vi "Open Running VI MHLC.vi"(8 "error in (no error)":errorcluster, 10 "Data in":variant, 11 "AppMgr in":refnum<class "Application Manager.lvclass">) -> (0 "error out":errorcluster, 3 "AppMgr out":refnum<class "Application Manager.lvclass">)   [LabVIEW 2017, in "Application Manager.lvclass"]
doc: "Open the Front Panel of the Main VI of the selected Worker's running clone"
uses:
  Application Manager.lvclass
  rqp_Open Running VI.ctl
  Common VIs/DC_UID.ctl
  Application Manager.lvclass/Application Manager.ctl
  rsp_Show Worker Block Diagram.ctl
  <vilib>/Utility/error.llb/Error Cluster From Error Code.vi
  <vilib>/ErrorRing/Error Ring.xnode
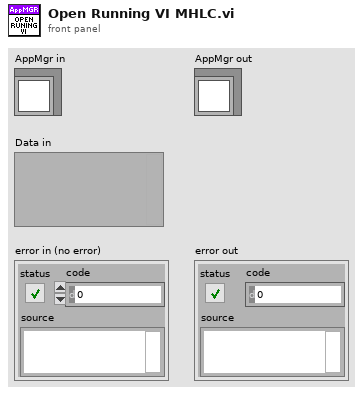
[diagram p1: front panel]
types:
  T1 = typedef "Application Manager.lvclass/rqp_Open Running VI.ctl" = cluster{"DC_UID":T2, "Worker ID":string}
  T2 = typedef "DC_UID.ctl" = string
  T3 = typedef "Application Manager.lvclass/Debug Client Data.ctl" = cluster{"DC_UID":T2, "IP Address":string, "Worker Data":T4[], "Connected":bool}
  T4 = typedef "Application Manager.lvclass/Worker Data.ctl" = cluster{"ID":string, "VI Ref":refnum<vi>, "VI Path":path, "CloneID":string, "Type":T5, "Worker Status":string}
  T5 = typedef "Workers.lvlib/Worker.lvclass/Worker Type.ctl" = enum16{"SL", "DL"}
  T6 = typedef "Application Manager.lvclass/rsp_Show Worker Block Diagram.ctl" = cluster{"DC_UID":T2, "VI Path":path, "VI Ref":refnum<vi>}
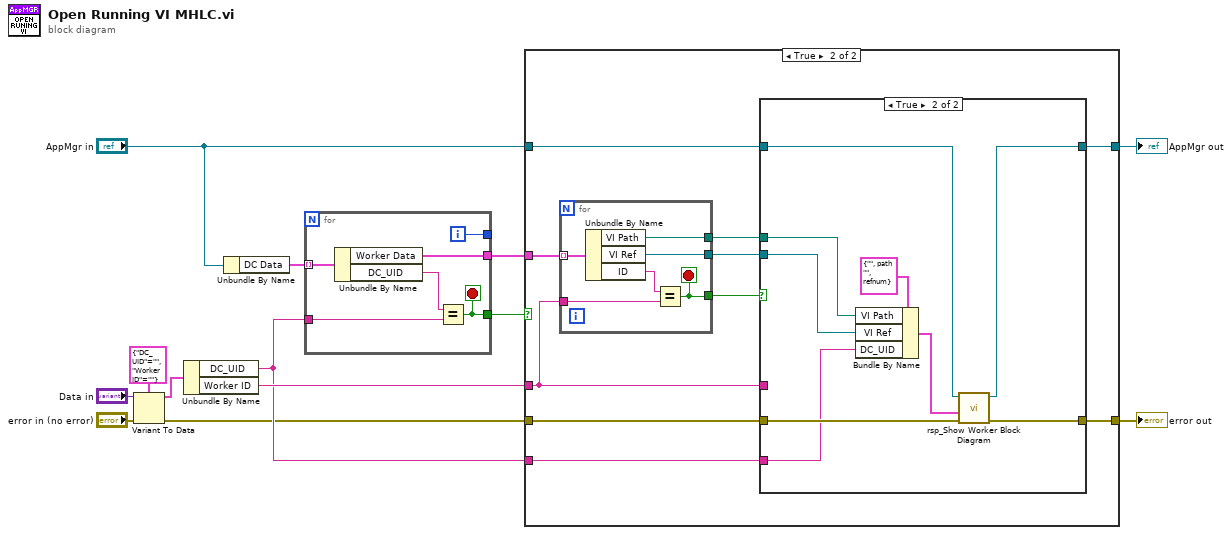
[diagram p0: block diagram]
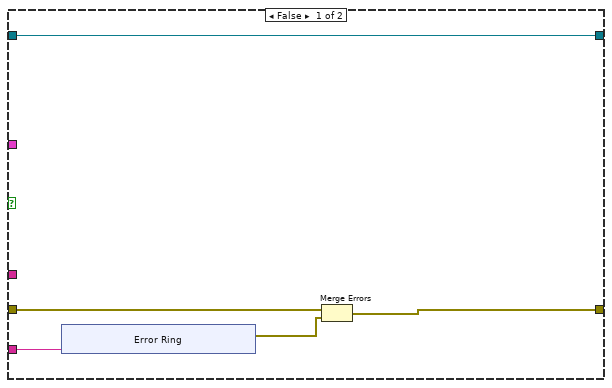
[diagram p2: hidden frame]
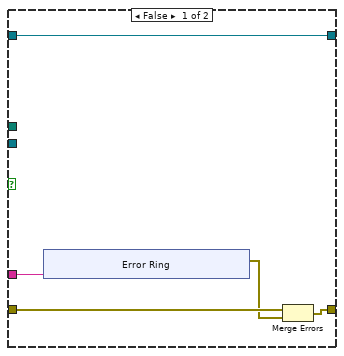
[diagram p3: hidden frame]
diagram:
  n1 = Variant To Data(error in="error in (no error)", type=T1 {"DC_UID"="", "Worker ID"=""} ("Data"), Variant="Data in") -> (data=w4:T1, error out=w8:errorcluster)
  n2 = Unbundle By Name(w4) -> ("DC_UID"=w11:T2, "Worker ID"=w13:string)
  n3 = Unbundle By Name("AppMgr in") -> ("DC Data"=w5:T3[])
  n4 = for {
    tunnel: w5 -> [w16] mode=indexing
    tunnel: [w18] -> w10
    tunnel: [w17] -> _
    tunnel: [w14] -> w12
    tunnel: w11 -> [w15]
    i -> [w17]
    stop <- w18 stop-if-true
    n5 = Unbundle By Name(w16) -> ("Worker Data"=w14:T4[], "DC_UID"=w19:T2)
    n6 = Equal?(x=w19, y=w15) -> (x = y?=w18:bool)
  }
  n7 = case shown="True" w10 {
    tunnel: "AppMgr in" -> [w24 w38]
    tunnel: [w24 w37] -> w7
    tunnel: w8 -> [w23 w41]
    tunnel: [w22 w39] -> w9
    tunnel: w11 -> [w20 w36]
    tunnel: w12 -> [_ w40]
    tunnel: w13 -> [_ w33]
    frame False {
      n8 = xnode "Error Ring"("parameter 0"=w20) -> ("error out"=w21:errorcluster)
      n9 = Merge Errors(w23, w21) -> (w22:errorcluster)
    }
    frame True {
      n10 = for {
        tunnel: w40 -> [w68] mode=indexing
        tunnel: w33 -> [w66]
        tunnel: [w65] -> w32
        tunnel: [w64] -> w34
        tunnel: [w63] -> w35
        stop <- w65 stop-if-true
        n11 = Unbundle By Name(w68) -> ("VI Path"=w64:path, "VI Ref"=w63:refnum<vi>, "ID"=w67:string)
        n12 = Equal?(x=w67, y=w66) -> (x = y?=w65:bool)
      }
      n13 = case shown="True" w32 {
        tunnel: w41 -> [w46 w62]
        tunnel: [w45 w61] -> w39
        tunnel: w38 -> [w44 w60]
        tunnel: [w44 w59] -> w37
        tunnel: w36 -> [_ w56]
        tunnel: w35 -> [_ w55]
        tunnel: w34 -> [_ w54]
        tunnel: w33 -> [w42 _]
        frame False {
          n14 = xnode "Error Ring"("parameter 0"=w42) -> ("error out"=w43:errorcluster)
          n15 = Merge Errors(w46, w43) -> (w45:errorcluster)
        }
        frame True {
          n16 = Bundle By Name(cluster=T6 {"DC_UID"="", "VI Path"=path "", "VI Ref"=refnum} ("Data in"), "VI Path"=w54, "VI Ref"=w55, "DC_UID"=w56) -> (w57:T6)
          n17 = call "rsp_Show Worker Block Diagram.vi"("error in"=w62, "Data in"=w57, "Application Manager in"=w60) -> ("error out"=w61:errorcluster, "dup Application Manager out"=w59:refnum<class "Application Manager.lvclass">)  [unwired: 7 in]
        }
      }
    }
  }
  "error out" <- w9
  "AppMgr out" <- w7
